vi "ReadBAESdataFromFile.vi"(0 "file path":path) -> (1 "WaveLengths":dbl[](array[numeric]), 2 "Number Of Sizes":dbl, 3 "Extinction":dbl[][](array[numeric]), 4 "ExtinctionUncertainty":dbl[][](array[numeric]), 5 "SizeParameter":dbl[][](array[numeric]), 6 "GeometricCrossSection":dbl[](array[numeric]))   [LabVIEW 2011]
uses:
  <vilib>/Platform/storage/lvStorage.llb/_openStorageWithRootAutoDetect.vi
  <vilib>/Platform/storage/lvStorage.llb/xStorage/xStorageSupp/ErrorOut.vi
  <vilib>/Platform/storage/lvStorage.llb/_queryPropDateTime.vi
  <vilib>/Platform/storage/lvStorage.llb/_queryGenericObjects.vi
  <vilib>/Platform/storage/lvStorage.llb/_loadAllDouble.vi
  <vilib>/Platform/storage/Storage.llb/Get Object Info.vi
  <vilib>/Platform/storage/Storage.llb/__closeStorageFromObject.vi
  <vilib>/imath/engines/lvmath2/RunTimeEngine/ErrorHandling/NIMS_Finalize Error.vi
  <vilib>/imath/engines/lvmath2/RunTimeEngine/Managers/WorkSpace/UID Generator.vi
  <vilib>/imath/engines/lvmath2/RunTimeEngine/VariableToken/Read/NIMS_Get Elements - SorM(_,$) - Check.vi
  <instcachedir>/0/NIMS_Get Elements - SorM(_,$) - Check_3B494CC2A76E49EA8E6F8F732E2632C3.lvgen/NIMS_Get Elements - SorM(_,$) - Check_3B494CC2A76E49EA8E6F8F732E2632C3_000.vi
  <vilib>/imath/engines/lvmath2/RunTimeEngine/BuiltInFunctions/length/NIMS_length(GV).vi
  <instcachedir>/0/NIMS_length(GV)_08A3D13377FD4E4B96F5795FBF3698FA.lvgen/NIMS_length(GV)_08A3D13377FD4E4B96F5795FBF3698FA_000.vi
  <vilib>/imathl/engines/lvmath/Functions/Error Handling/Create Error.vi
  <vilib>/imath/engines/lvmath2/RunTimeEngine/Managers/SymbolTable/Clear UID.vi
  <vilib>/imath/engines/lvmath2/RunTimeEngine/NodeEndStatement/NIMS_NodeEndStatement_Output.vi
  <instcachedir>/0/NIMS_NodeEndStatement_Output_53EC0D466D134D7ABD903AC30B43404B.lvgen/NIMS_NodeEndStatement_Output_53EC0D466D134D7ABD903AC30B43404B_005.vi
  <instcachedir>/0/NIMS_NodeEndStatement_Output_53EC0D466D134D7ABD903AC30B43404B.lvgen/NIMS_NodeEndStatement_Output_53EC0D466D134D7ABD903AC30B43404B_001.vi
  <instcachedir>/0/NIMS_NodeEndStatement_Output_53EC0D466D134D7ABD903AC30B43404B.lvgen/NIMS_NodeEndStatement_Output_53EC0D466D134D7ABD903AC30B43404B_002.vi
  <vilib>/imath/engines/lvmath2/RunTimeEngine/RangeToken/NIMS_Range.vi
  <instcachedir>/0/NIMS_Range_0B7635FB69F84E19AA68E7FF959DF37C.lvgen/NIMS_Range_0B7635FB69F84E19AA68E7FF959DF37C_001.vi
  <vilib>/imath/engines/lvmath2/RunTimeEngine/VariableToken/Read/NIMS_Get Elements - SorM(_,_) - Check - Check(_).vi
  <instcachedir>/0/NIMS_Get Elements - SorM(_,_) - Check - Check(_)_B78B880141DE464ABBC753BC43E627FC.lvgen/NIMS_Get Elements - SorM(_,_) - Check - Check(_)_B78B880141DE464ABBC753BC43E627FC_009.vi
  <vilib>/imath/engines/lvmath2/RunTimeEngine/ErrorHandling/NIMS_Create Error From Enums.vi
  <vilib>/imath/engines/lvmath2/RunTimeEngine/RangeToken/NIMS_Range_R2.vi
  <vilib>/imath/engines/lvmath2/RunTimeEngine/VariableToken/Read/NIMS_Get Elements - SorM(_,_) - Check - Check.vi
  <instcachedir>/0/NIMS_Get Elements - SorM(_,_) - Check - Check_DA1E252EAB634D989357E7C72E8137F5.lvgen/NIMS_Get Elements - SorM(_,_) - Check - Check_DA1E252EAB634D989357E7C72E8137F5_006.vi
  <vilib>/imath/engines/lvmath2/RunTimeEngine/BuiltInFunctions/repeatmx/NIMS_repeatmx(GM, I32, I32).vi
  <instcachedir>/0/NIMS_repeatmx(GM, I32, I32)_8C2ED2EBCBCE41FC8E83AC0E124C0986.lvgen/NIMS_repeatmx(GM, I32, I32)_8C2ED2EBCBCE41FC8E83AC0E124C0986_000.vi
  <vilib>/imath/engines/lvmath2/RunTimeEngine/ArithmeticOperatorToken/NIMS_ArithmeticOperator_rightdiv.vi
  <instcachedir>/0/NIMS_ArithmeticOperator_rightdiv_85C5B8074732470A99000A2C3876C445.lvgen/NIMS_ArithmeticOperator_rightdiv_85C5B8074732470A99000A2C3876C445_004.vi
  <vilib>/imath/engines/lvmath2/RunTimeEngine/RunTimeType/NIMS_RunTimeType_From StrictType (excl LVString).vi
  <instcachedir>/0/NIMS_RunTimeType_From StrictType (excl LVString)_46AE8B54A11948F0BCCEB8091EE7AA4C.lvgen/NIMS_RunTimeType_From StrictType (excl LVString)_46AE8B54A11948F0BCCEB8091EE7AA4C_000.vi
  <vilib>/imath/engines/lvmath2/RunTimeEngine/LocalVariableDefStatement/MC_LocalVariableDefStatement_Display.vi
  <instcachedir>/0/NIMS_Get Elements - SorM(_,_) - Check - Check(_)_B78B880141DE464ABBC753BC43E627FC.lvgen/NIMS_Get Elements - SorM(_,_) - Check - Check(_)_B78B880141DE464ABBC753BC43E627FC_010.vi
  <vilib>/Platform/storage/lvStorage.llb/xStorage/Open Data Storage/Open Data Storage.xnode
  <vilib>/Platform/storage/lvStorage.llb/xStorage/Read Data/Read Data.xnode
  <vilib>/Platform/storage/lvStorage.llb/xStorage/Close Data Storage/Close Data Storage.xnode
  <vilib>/imath/engines/lvmath2/RunTimeEngine/Managers/SymbolTable/NIMS_WorkSpace.lvlib
panel:
  out "Signal":dbl[][](array[numeric])
  in  "Slide":i16(slide) scale=0.0..100.0
  out "Extinction Graph":cluster{"Extinction":dbl[], "Sizes":dbl[]}[](graph)
  out "error out":errorcluster
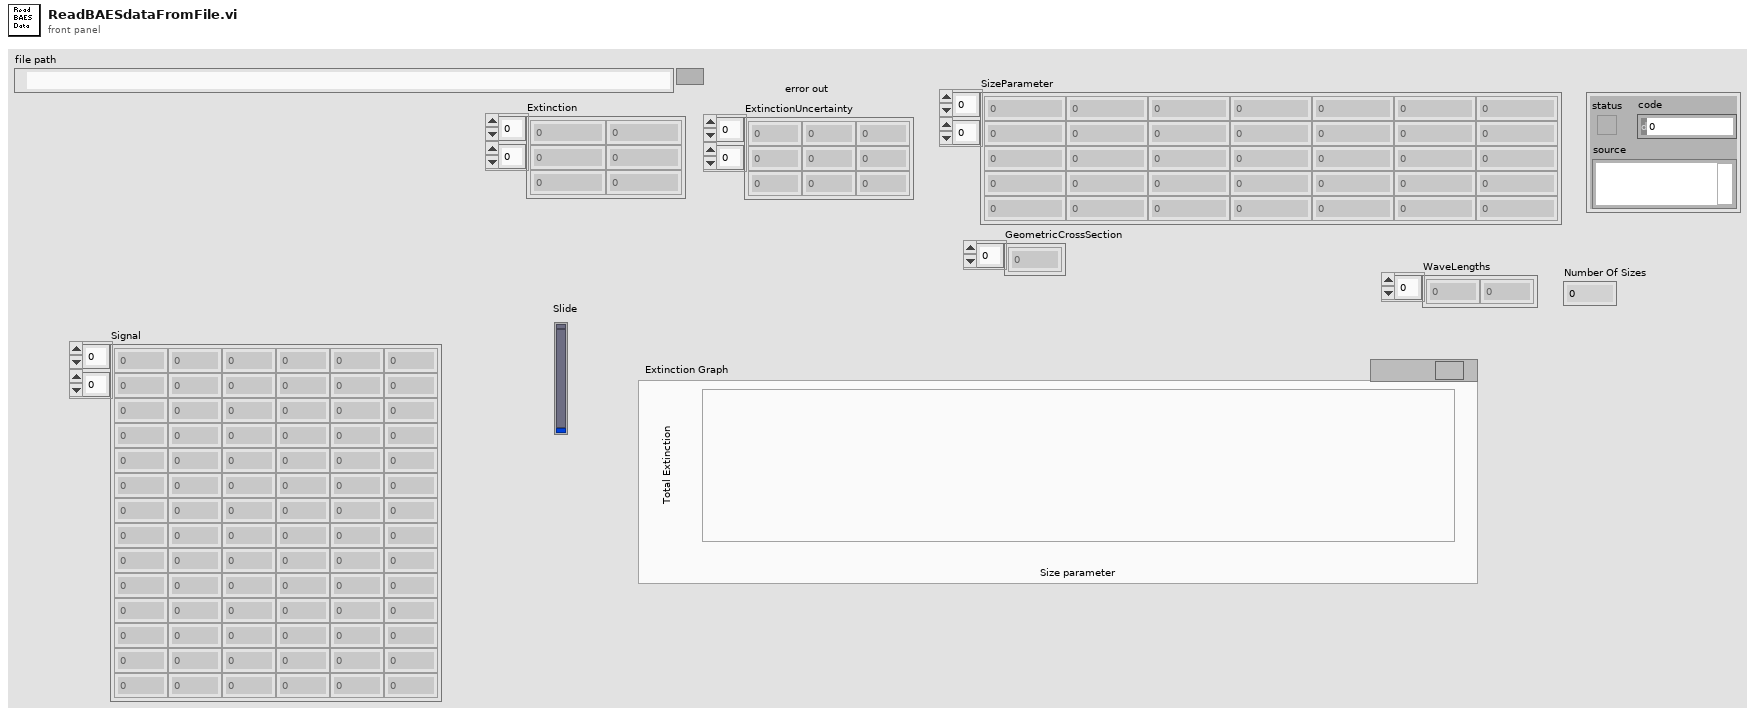
[diagram p1: front panel]
types:
  T1 = enum16{"open", "open or create", "create or replace", "create", "open (read only)"}
  T2 = cluster{"SizeParameter":dbl[], "Extinction":dbl[]}
  T3 = cluster{"SizeParameter":dbl[], "Extinction":dbl[]}[]
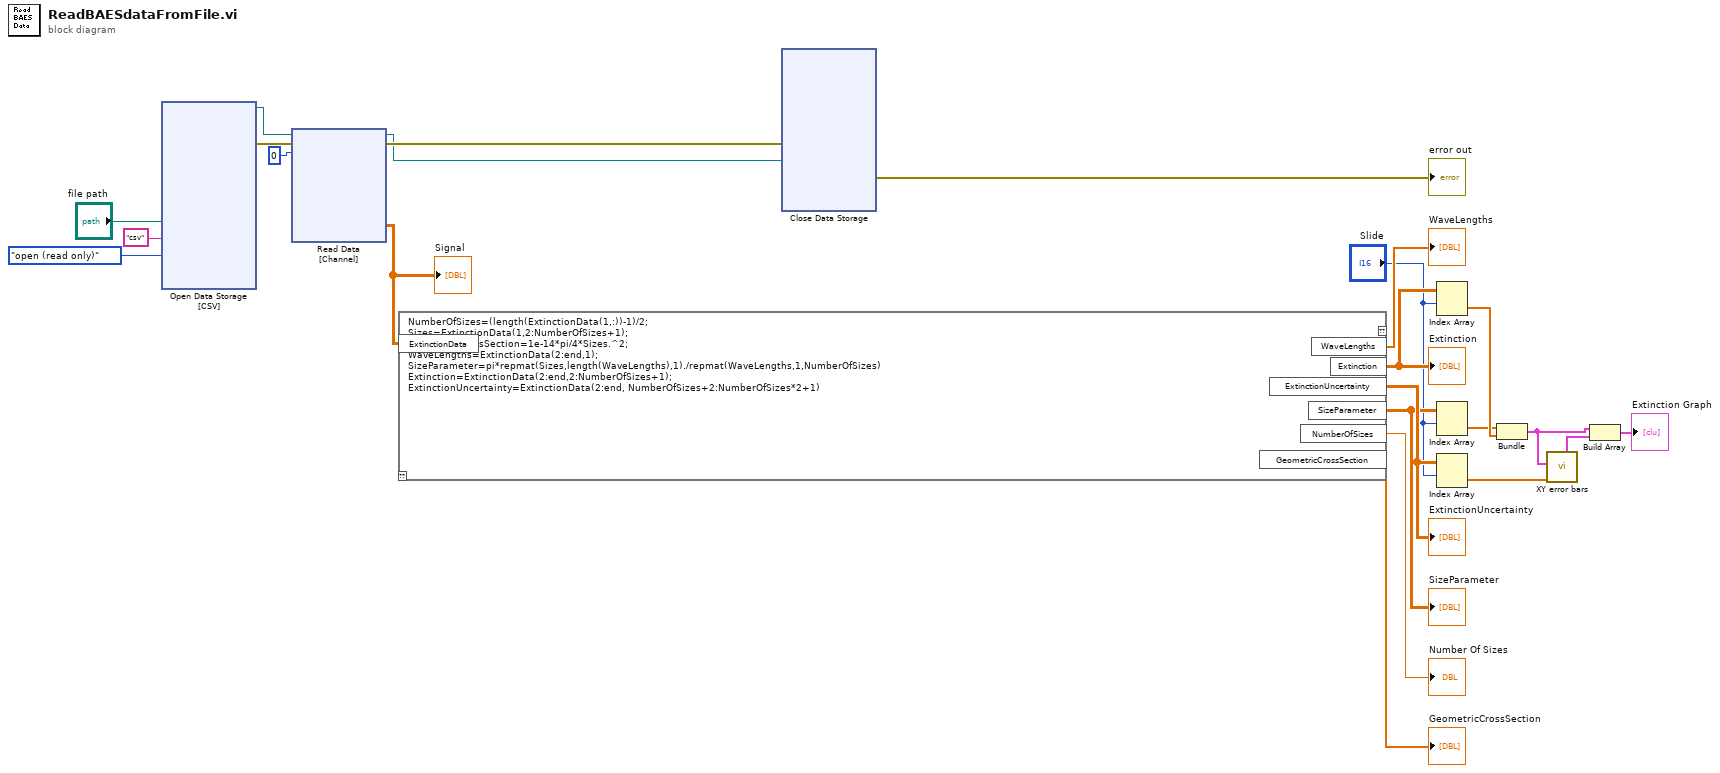
[diagram p0: block diagram]
diagram:
  n1 = xnode "Open Data Storage\n[CSV]"("file path"="file path", "DataPlugin name"="csv", "function (open:0)"=T1."open (read only)") -> ("storage refnum (file)"=w23:refnum<k20>, "error out"=w22:errorcluster)  [unwired: 2 in, 1 out]
  n2 = xnode "Read Data\n[Channel]"("storage refnum (file)"=w23, "error in"=w22, "index"=0) -> ("Signal"=w5:dbl[][], "storage refnum (file) out"=w17:refnum<k20>, "error out"=w21:errorcluster)  [unwired: 1 in, 1 out]
  "Signal" <- w5
  n3 = mathscript code="NumberOfSizes=(length(ExtinctionData(1,:))-1)/2;\nSizes=ExtinctionData(1,2:NumberOfSizes+1);\nGeometricCrossSection=1e-14*pi/4*Sizes.^2;\nWaveLengths=ExtinctionData(2:end,1);\nSizeParameter=pi*repmat(Sizes,length(WaveLengths),1)./repmat(WaveLengths,1,NumberOfSizes)\nExtinction=ExtinctionData(2:end,2:NumberOfSizes+1);\nExtinctionUncertainty=ExtinctionData(2:end, NumberOfSizes+2:NumberOfSizes*2+1)"("ExtinctionData"=w5) -> ("WaveLengths"=→"WaveLengths":dbl[], "Extinction"=w15:dbl[][], "ExtinctionUncertainty"=w14:dbl[][], "SizeParameter"=w8:dbl[][], "NumberOfSizes"=→"Number Of Sizes":dbl, "GeometricCrossSection"=→"GeometricCrossSection":dbl[])  [unwired: 1 in, 1 out]
  "Extinction" <- w15
  "ExtinctionUncertainty" <- w14
  "SizeParameter" <- w8
  n4 = xnode "Close Data Storage\n"("error in (no error)"=w21, "storage refnum (file)"=w17) -> ("error out"=→"error out":errorcluster)  [unwired: 1 out]
  n5 = Index Array(array=w15, index (row)="Slide") -> (element=w9:dbl[])  [unwired: 1 in]
  n6 = Index Array(array=w8, index (row)="Slide") -> (element=w6:dbl[])  [unwired: 1 in]
  n7 = Index Array(array=w14, index (row)="Slide") -> (element=w13:dbl[])  [unwired: 1 in]
  n8 = Bundle("SizeParameter"=w6, "Extinction"=w9) -> (w12:T2)  [unwired: 1 in]
  n9 = call "XY error bars.vi"("XY plot"=w12, "Yerror"=w13) -> ("Y error bars"=w11:cluster{dbl[], dbl[]})  [unwired: 6 in, 2 out]
  n10 = Build Array(w12, w11) -> (→"Extinction Graph":T3)
